vi "ADC500_CFG.vi"(0 "TCP Network Connection in":refnum<k5>, 1 "OUTV":bool, 3 "DDR":bool, 4 "DCLK_RST":bool, 5 "error in (no error)":errorcluster, 6 "Full Scale Range":bool, 7 "ON":bool, 10 "CAL_DLY":bool, 11 "LED 0":bool, 12 "CAL":bool, 13 "LED 1":bool) -> (14 "TCP Network Connection out":refnum<k5>, 15 "ADC500_STATUS":u8[](array[numeric]), 17 "ADC500_CFG":u32, 19 "error out":errorcluster)   [LabVIEW 2019]
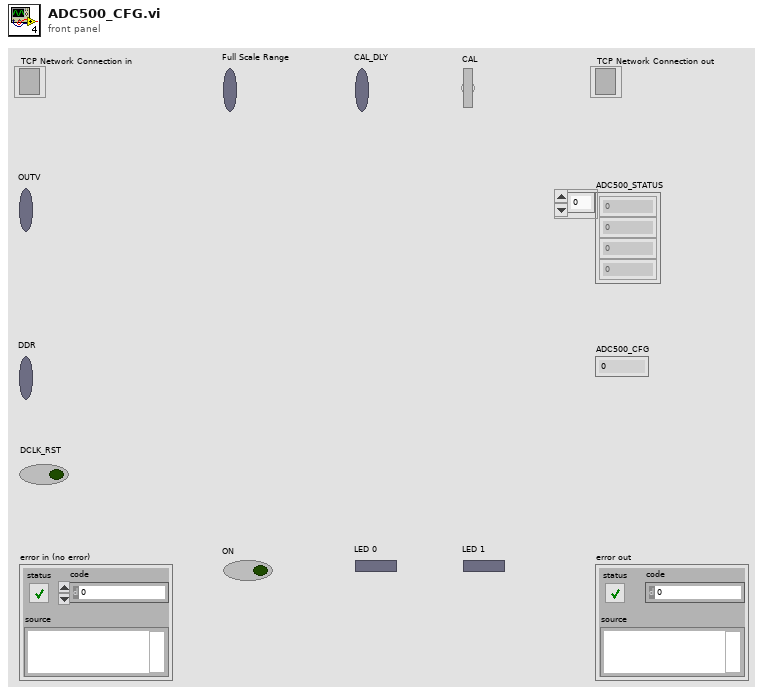
[diagram p1: front panel]
types:
  T1 = enum16{"big-endian, network order", "native, host order", "little-endian"}
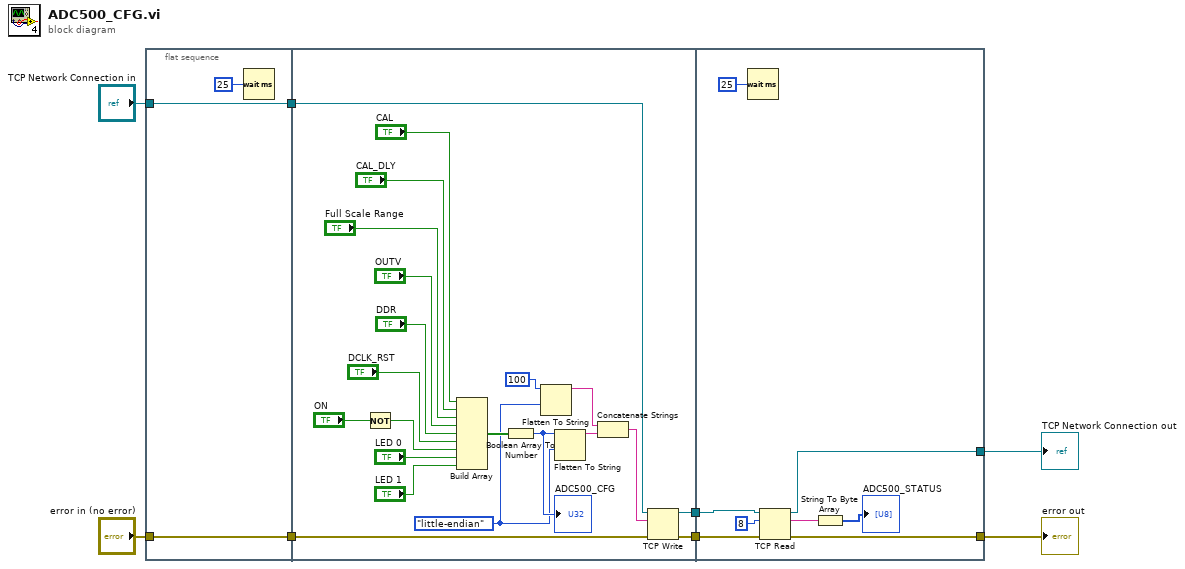
[diagram p0: block diagram]
diagram:
  n1 = flat-sequence {
    tunnel: [w10] -> w4
    tunnel: [w11] -> w3
    tunnel: "error in (no error)" -> [w11]
    tunnel: "TCP Network Connection in" -> [w10]
    tunnel: w4 -> [w22]
    tunnel: w3 -> [w21]
    tunnel: [w20] -> w2
    tunnel: [w19] -> w1
    tunnel: [w37] -> w6
    tunnel: [w38] -> w5
    tunnel: w2 -> [w40]
    tunnel: w1 -> [w39]
    frame #0 {
      n2 = Wait (ms)(milliseconds to wait=u32 25) -> ()  [unwired: 1 out]
    }
    frame #1 {
      w15 = T1."little-endian" ("byte order (0:big-endian, network order)")
      n3 = Not(x="ON") -> (.not. x?=w23:bool)
      n4 = Build Array("CAL", "CAL_DLY", "Full Scale Range", "OUTV", "DDR", "DCLK_RST", w23, "LED 0", "LED 1") -> (w17:bool[])
      n5 = Boolean Array To Number(Boolean array=w17) -> (number=w18:u32)
      "ADC500_CFG" <- w18
      n6 = Flatten To String(anything=u32 100 ("element"), byte order (0:big-endian, network order)=w15) -> (data string=w13:string)  [unwired: 2 in, 2 out]
      n7 = Flatten To String(anything=w18, byte order (0:big-endian, network order)=w15) -> (data string=w16:string)  [unwired: 2 in, 2 out]
      n8 = Concatenate Strings(w13, w16) -> (w12:string)
      n9 = TCP Write(connection ID=w22, data in=w12, error in (no error)=w21) -> (connection ID out=w20:refnum<k5>, error out=w19:errorcluster)  [unwired: 1 in, 1 out]
    }
    frame #2 {
      n10 = Wait (ms)(milliseconds to wait=u32 25) -> ()  [unwired: 1 out]
      n11 = TCP Read(connection ID=w40, bytes to read=8, error in (no error)=w39) -> (connection ID out=w38:refnum<k5>, data out=w34:string, error out=w37:errorcluster)  [unwired: 2 in]
      n12 = String To Byte Array(string=w34) -> (unsigned byte array=→"ADC500_STATUS":u8[])
    }
  }
  "error out" <- w6
  "TCP Network Connection out" <- w5
